vi "InitPort.vi"(8 "error in (no error)":errorcluster, 11 "VISA resource name":refnum<visa-resource-name>) -> (0 "error out":errorcluster, 3 "VISA resource name out":refnum<visa-resource-name>)   [LabVIEW 2009]
uses:
  <vilib>/Instr/_visa.llb/VISA Set IO Buffer Mask.ctl
  <vilib>/Instr/_visa.llb/VISA Flush IO Buffer Mask.ctl
  <vilib>/Instr/_visa.llb/VISA Configure Serial Port (Instr).vi
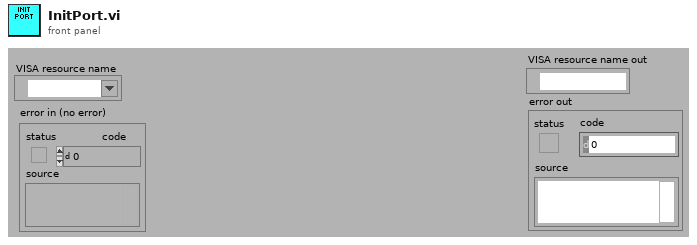
[diagram p1: front panel]
types:
  T1 = typedef "VISA Flush IO Buffer Mask.ctl" = u16
  T2 = typedef "VISA Set IO Buffer Mask.ctl" = u16
  T3 = cluster{"Frame Byte":u8, "EscapeByte":u8, "XOR Byte":u8}
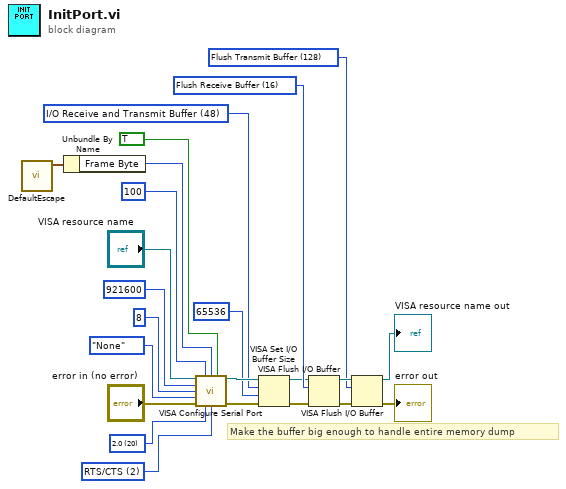
[diagram p0: block diagram]
diagram:
  w5 = T1 128 items=["Flush Receive Buffer"=16, "Write Transmit Buffer to Device"=32, "Flush Receive Buffer (No I/O)"=64, "Flush Transmit Buffer"=128] ("Mask")
  w10 = T1 16 items=["Flush Receive Buffer"=16, "Write Transmit Buffer to Device"=32, "Flush Receive Buffer (No I/O)"=64, "Flush Transmit Buffer"=128] ("Mask")
  w12 = T2 48 items=["I/O Receive Buffer"=16, "I/O Transmit Buffer"=32, "I/O Receive and Transmit Buffer"=48] ("Mask")
  w20 = u16 2 items=["None", "XON/XOFF", "RTS/CTS", "XON/XOFF & RTS/CTS", "DTR/DSR", "XON/XOFF & DTR/DSR"] ("flow control (0:none)")
  w21 = u16 20 items=["1.0"=10, "1.5"=15, "2.0"=20] ("stop bits (10: 1 bit)")
  # "Make the buffer big enough to handle entire memory dump"
  n1 = call "DefaultEscape.vi"() -> ("EscapePattern"=w4:T3)  [unwired: 11 in]
  n2 = Unbundle By Name(w4) -> ("Frame Byte"=w3:u8)
  n3 = call-poly "VISA Configure Serial Port"("VISA resource name"="VISA resource name", "timeout (10sec)"=u32 100, "termination char\n(0xA = '\\n' = LF)"=w3, "Enable Termination\nChar (T)"=TRUE ("Enable Termination\nChar (T)"), "baud rate (9600)"=u32 921600, "data bits (8)"=u16 8, "parity (0:none)"=enum16{"None", "Odd", "Even", "Mark", "Space"}."None", "error in (no error)"="error in (no error)", "stop bits (10: 1 bit)"=w21, "flow control (0:none)"=w20) -> ("VISA resource name out"=w14:refnum<visa-resource-name>, "error out"=w13:errorcluster)  [unwired: 4 in]
  n4 = VISA Set I/O Buffer Size(VISA resource name=w14, mask (16)=w12, size (4096)=u32 65536, error in (no error)=w13) -> (VISA resource name out=w2:refnum<visa-resource-name>, error out=w1:errorcluster)
  n5 = VISA Flush I/O Buffer(VISA resource name=w2, mask (16)=w10, error in (no error)=w1) -> (VISA resource name out=w6:refnum<visa-resource-name>, error out=w9:errorcluster)
  n6 = VISA Flush I/O Buffer(VISA resource name=w6, mask (16)=w5, error in (no error)=w9) -> (VISA resource name out=→"VISA resource name out":refnum<visa-resource-name>, error out=→"error out":errorcluster)
